vi "globalSetUp.vi"(8 "error in (no error)":errorcluster, 11 "testcase-CSMAddonLoopSupport.lvclass in":refnum<class "testcase-CSMAddonLoopSupport.lvclass">) -> (0 "error out":errorcluster, 3 "testcase-CSMAddonLoopSupport.lvclass out":refnum<class "testcase-CSMAddonLoopSupport.lvclass">)   [LabVIEW 2017, in "testcase-CSMAddonLoopSupport.lvclass"]
uses:
  testcase-CSMAddonLoopSupport.lvclass
  <vilib>/addons/_JKI Toolkits/VI Tester/TestCase.llb/TestCase.lvclass
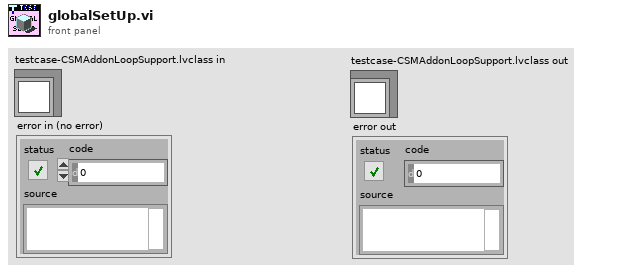
[diagram p1: front panel]
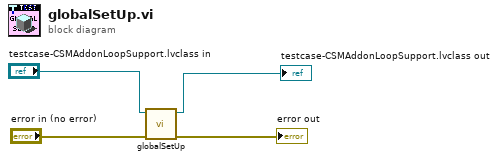
[diagram p0: block diagram]
diagram:
  n1 = call-parent "globalSetUp.vi"("error in (no error)"="error in (no error)", "TestCase in"="testcase-CSMAddonLoopSupport.lvclass in") -> ("error out"=→"error out":errorcluster, "TestCase out"=→"testcase-CSMAddonLoopSupport.lvclass out":refnum<class "testcase-CSMAddonLoopSupport.lvclass">)  [unwired: 8 in]
